vi "Read Configuration Parameters.vi"(8 "error in (no error)":errorcluster, 10 "refnum":T1, 11 "VacuumLines Configuration in":refnum<class "VacuumLines Configuration.lvclass">) -> (0 "error out":errorcluster, 2 "refnum out":T1, 3 "VacuumLines Configuration out":refnum<class "VacuumLines Configuration.lvclass">)   [LabVIEW 2016, in "Hardware.lvlib" / "VacuumLine.lvlib" / "VacuumLines Configuration.lvclass"]
uses:
  <userlib>/Common Components/Hardware/Abstract System/VacuumLine/VacuumLines Configuration/VacuumLines Configuration.lvclass
  <vilib>/Utility/config.llb/Config Data RefNum.ctl
  <userlib>/Common Components/Hardware/Abstract System/VacuumLine/VacuumLines Configuration/VacuumLines Configuration.lvclass/VacuumLines Configuration.ctl
  <userlib>/Common Components/Hardware/Abstract System/VacuumLine/VacuumLine Config/VacuumLine Configuration.lvclass/VacuumLine Configuration.ctl
  <userlib>/Common Components/Hardware/Abstract System/VacuumLine/VacuumLines/VacuumLines.lvclass/VacuumLines.ctl
  <userlib>/Common Components/UserPwd DB/UserPwd DB Config/UserPwd DB Configuration.lvclass/UserPwd DB Configuration.ctl
  <userlib>/Common Components/Hardware/Abstract System/VacuumLine/VacuumLine Config/VacuumLine Configuration.lvclass
  <userlib>/Common Components/Hardware/Abstract System/VacuumLine/VacuumLines/VacuumLines.lvclass
  <userlib>/Common Components/Hardware/GaugeController/GaugeController/GaugeController.lvclass
  <userlib>/Common Components/UserPwd DB/UserPwd DB Config/UserPwd DB Configuration.lvclass
  <vilib>/Utility/config.llb/NI_LVConfig.lvlib
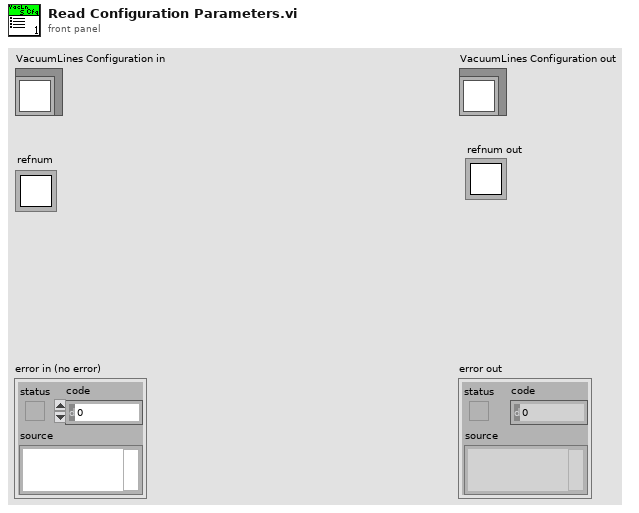
[diagram p1: front panel]
types:
  T1 = typedef "NI_LVConfig.lvlib/Config Data RefNum.ctl" = refnum<k1>
  T2 = cluster{"Conflict Zones":string, "More Valves":string, "Pressure Display":string, "Temperature":string}
  T3 = typedef "Hardware.lvlib/VacuumLine.lvlib/VacuumLines.lvclass/Conflict Zone.ctl" = cluster{"Conflict Zone":cluster{"1":cluster{"Label":string, "from":dbl, "to":dbl, "buffer":dbl}, "2":cluster{"Label":string, "from":dbl, "to":dbl, "buffer":dbl}}}
  T4 = typedef "Hardware.lvlib/VacuumLine.lvlib/VacuumLines.lvclass/LogicOut.ctl" = cluster{"Label":string, "LogicIO Module":string, "Pin#":u8}
  T5 = typedef "Hardware.lvlib/VacuumLine.lvlib/VacuumLines.lvclass/Gauge Param.ctl" = cluster{"label":string, "Gauge Controller":string, "Channel":enum16{"1", "2", "3", "4", "5", "6", "7", "8"}, "Threshold":dbl}
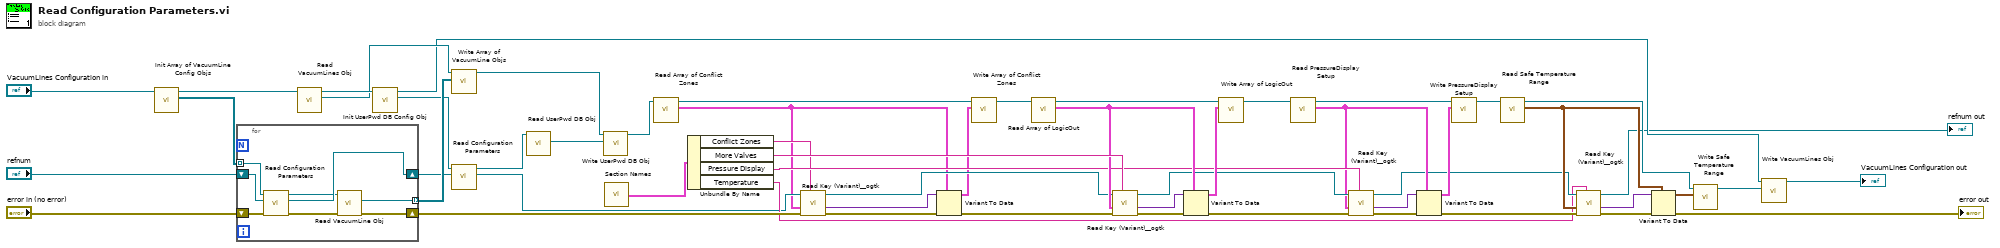
[diagram p0: block diagram]
diagram:
  n1 = call <userlib>:"Init Array of VacuumLine Config Objs.vi"("VacuumLines Configuration in"="VacuumLines Configuration in") -> ("Array of VacuumLine Config Objs"=w47:refnum<class "VacuumLine Configuration.lvclass">[], "VacuumLines Configuration out"=w48:refnum<class "VacuumLines Configuration.lvclass">)  [unwired: 8 in, 1 out]
  n2 = for {
    tunnel: w47 -> [w59] mode=indexing
    shift-right: [w58] -> w52
    shift-left: "error in (no error)" -> [w63]
    shift-right: [w60] -> w14
    shift-left: "refnum" -> [w61]
    tunnel: [w56] -> w50 mode=indexing
    n3 = call-dynamic "Read Configuration Parameters.vi"("error in (no error)"=w63, "refnum"=w61, "VacuumLine Configuration in"=w59) -> ("error out"=w62:errorcluster, "refnum out"=w60:T1, "VacuumLine Configuration out"=w57:refnum<class "VacuumLine Configuration.lvclass">)  [unwired: 6 in]
    n4 = call <userlib>:"Read VacuumLine Obj.vi"("error in (no error)"=w62, "VacuumLine Configuration in"=w57) -> ("error out"=w58:errorcluster, "Hardware.lvlib:VacuumLine.lvlib:VacuumLine.lvclass"=w56:refnum<class "VacuumLine.lvclass">)  [unwired: 7 in, 1 out]
  }
  n5 = call <userlib>:"Read VacuumLines Obj.vi"("VacuumLines Configuration in"=w48) -> ("Hardware.lvlib:VacuumLine.lvlib:VacuumLines.lvclass"=w38:refnum<class "VacuumLines.lvclass">, "VacuumLines Configuration out"=w54:refnum<class "VacuumLines Configuration.lvclass">)  [unwired: 8 in, 1 out]
  n6 = call <userlib>:"Init UserPwd DB Config Obj.vi"("VacuumLines Configuration in"=w54) -> ("UserPwd DB Configuration Obj"=w27:refnum<class "UserPwd DB Configuration.lvclass">, "VacuumLines Configuration out"=w28:refnum<class "VacuumLines Configuration.lvclass">)  [unwired: 8 in, 1 out]
  n7 = call <userlib>:"Write Array of VacuumLine Objs.vi"("Array of VacuumLine Objs"=w50, "VacuumLines in"=w38) -> ("VacuumLines out"=w49:refnum<class "VacuumLines.lvclass">)  [unwired: 9 in]
  n8 = call-dynamic "Read Configuration Parameters.vi"("refnum"=w14, "UserPwd DB Configuration in"=w27) -> ("refnum out"=w9:T1, "UserPwd DB Configuration out"=w24:refnum<class "UserPwd DB Configuration.lvclass">)  [unwired: 7 in, 1 out]
  n9 = call <userlib>:"Read UserPwd DB Obj.vi"("UserPwd DB Configuration in"=w24) -> ("UserPwd DB.lvlib:UserPwd DB.lvclass"=w12:refnum<class "UserPwd DB.lvclass">)  [unwired: 9 in, 1 out]
  n10 = call <userlib>:"Write UserPwd DB Obj.vi"("UserPwd DB.lvlib:UserPwd DB.lvclass"=w12, "VacuumLines in"=w49) -> ("VacuumLines out"=w15:refnum<class "VacuumLines.lvclass">)  [unwired: 9 in]
  n11 = call <userlib>:"Section Names.vi"() -> ("Cluster"=w45:T2)
  n12 = call <userlib>:"Read Array of Conflict Zones.vi"("VacuumLines in"=w15) -> ("Array of Conflict Zones"=w3:T3[], "VacuumLines out"=w5:refnum<class "VacuumLines.lvclass">)  [unwired: 9 in]
  n13 = Unbundle By Name(w45) -> ("Conflict Zones"=w6:string, "More Valves"=w44:string, "Pressure Display"=w32:string, "Temperature"=w11:string)
  n14 = call <userlib>:"Read Key (Variant)__ogtk.vi"("section"=w6, "error in (no error)"=w52, "type"=w3, "refnum"=w9) -> ("error out"=w10:errorcluster, "key-value"=w4:variant, "refnum out"=w8:T1)  [unwired: 4 in, 1 out]
  n15 = Variant To Data(error in=w10, type=w3, Variant=w4) -> (data=w1:T3[], error out=w7:errorcluster)
  n16 = call <userlib>:"Write Array of Conflict Zones.vi"("Array of Conflict Zones"=w1, "VacuumLines in"=w5) -> ("VacuumLines out"=w2:refnum<class "VacuumLines.lvclass">)  [unwired: 9 in]
  n17 = call <userlib>:"Read Array of LogicOut.vi"("VacuumLines in"=w2) -> ("Array of LogicOut"=w40:T4[], "VacuumLines out"=w43:refnum<class "VacuumLines.lvclass">)  [unwired: 9 in]
  n18 = call <userlib>:"Read Key (Variant)__ogtk.vi"("section"=w44, "error in (no error)"=w7, "type"=w40, "refnum"=w8) -> ("error out"=w46:errorcluster, "key-value"=w41:variant, "refnum out"=w33:T1)  [unwired: 4 in, 1 out]
  n19 = Variant To Data(error in=w46, type=w40, Variant=w41) -> (data=w39:T4[], error out=w42:errorcluster)
  n20 = call <userlib>:"Write Array of LogicOut.vi"("Array of LogicOut"=w39, "VacuumLines in"=w43) -> ("VacuumLines out"=w37:refnum<class "VacuumLines.lvclass">)  [unwired: 9 in]
  n21 = call <userlib>:"Read PressureDisplay Setup.vi"("VacuumLines in"=w37) -> ("PressureDisplay Setup"=w31:T5[], "VacuumLines out"=w36:refnum<class "VacuumLines.lvclass">)  [unwired: 9 in]
  n22 = call <userlib>:"Read Key (Variant)__ogtk.vi"("section"=w32, "error in (no error)"=w42, "type"=w31, "refnum"=w33) -> ("error out"=w35:errorcluster, "key-value"=w30:variant, "refnum out"=w13:T1)  [unwired: 4 in, 1 out]
  n23 = Variant To Data(error in=w35, type=w31, Variant=w30) -> (data=w29:T5[], error out=w34:errorcluster)
  n24 = call <userlib>:"Write PressureDisplay Setup.vi"("PressureDisplay Setup"=w29, "VacuumLines in"=w36) -> ("VacuumLines out"=w25:refnum<class "VacuumLines.lvclass">)  [unwired: 9 in]
  n25 = call <userlib>:"Read Safe Temperature Range.vi"("VacuumLines in"=w25) -> ("Safe Temperature Range"=w18:cluster{"min":dbl, "max":dbl}, "VacuumLines out"=w23:refnum<class "VacuumLines.lvclass">)  [unwired: 9 in]
  n26 = call <userlib>:"Read Key (Variant)__ogtk.vi"("section"=w11, "error in (no error)"=w34, "type"=w18, "refnum"=w13) -> ("error out"=w21:errorcluster, "key-value"=w19:variant, "refnum out"=→"refnum out":T1)  [unwired: 4 in, 1 out]
  n27 = Variant To Data(error in=w21, type=w18, Variant=w19) -> (data=w17:cluster{"min":dbl, "max":dbl}, error out=→"error out":errorcluster)
  n28 = call <userlib>:"Write Safe Temperature Range.vi"("Safe Temperature Range"=w17, "VacuumLines in"=w23) -> ("VacuumLines out"=w22:refnum<class "VacuumLines.lvclass">)  [unwired: 9 in]
  n29 = call <userlib>:"Write VacuumLines Obj.vi"("Hardware.lvlib:VacuumLine.lvlib:VacuumLines.lvclass"=w22, "VacuumLines Configuration in"=w28) -> ("VacuumLines Configuration out"=→"VacuumLines Configuration out":refnum<class "VacuumLines Configuration.lvclass">)  [unwired: 8 in, 1 out]
